vi "CryoServer Add Channel.vi"(11 "value":T1) -> (3 "HK Item out":refnum<class "HK Item.lvclass">)   [LabVIEW 2024, in "CryoServer.lvclass"]
uses:
  CryoServer.lvclass
  CryoServer Channel Mapping.ctl
  hk-channel-class/hk-channel-class/HK Item/HK Item.lvclass
  hk-channel-class/hk-channel-class/HK Item/HK Channel Units and Setup.ctl
  hk-channel-class/hk-channel-class/HK Item/HK Channel enum Data Type.ctl
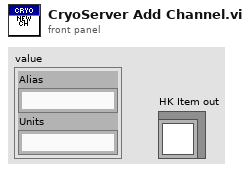
[diagram p1: front panel]
types:
  T1 = typedef "CryoServer Channel Mapping.ctl" = cluster{"Alias":string, "Units":string}
  T2 = typedef "HK Item.lvclass/HK Channel enum Data Type.ctl" = enum16{"Floating Point", "Integer", "Enum", "String", "Waveform", "File"}
  T3 = typedef "HK Item.lvclass/HK Channel Units and Setup.ctl" = cluster{"Unit Type":string, "Units":string, "Configuration":string, "Digits":i32, "Data Type":T2, "Exponential?":bool, "Source":string}
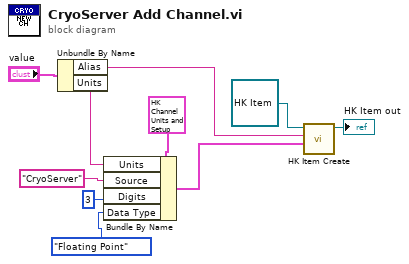
[diagram p0: block diagram]
diagram:
  n1 = Unbundle By Name("value") -> ("Alias"=w2:string, "Units"=w1:string)
  n2 = Bundle By Name(cluster=T3 {"Unit Type"="", "Units"="", "Configuration"="", "Digits"=0, "Data Type"=enum."Floating Point", "Exponential?"=FALSE, "Source"=""} ("Channel Setup"), "Units"=w1, "Source"="CryoServer", "Digits"=3, "Data Type"=HK_Channel_enum_Data_Type."Floating Point") -> (w9:T3)
  n3 = call-dynamic "HK Item Create.vi"("Channel Setup"=w9, "Name"=w2, "HK Item in"=refnum<class "HK Item.lvclass"> refnum) -> ("HK Item out"=→"HK Item out":refnum<class "HK Item.lvclass">)  [unwired: 7 in, 1 out]
